vi "Init Command Data.vi"() -> (1 "LBCB 2 Command Data":T1, 2 "LBCB 1 Command Data":T1)   [LabVIEW 2013]
uses:
  MixedMode/Target Data.ctl
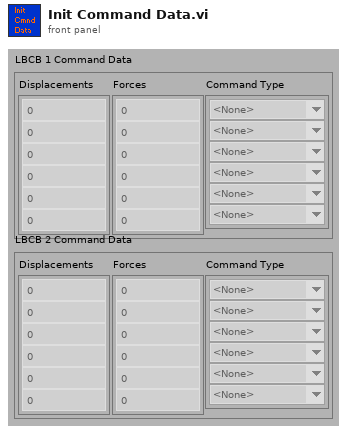
[diagram p1: front panel]
types:
  T1 = typedef "Target Data.ctl" = cluster{"Displacements":dbl[], "Command Type":enum16{"<None>", "Displacement", "Force"}[], "Forces":dbl[]}
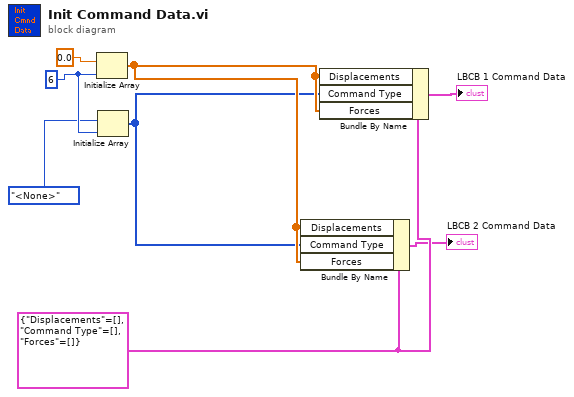
[diagram p0: block diagram]
diagram:
  w7 = 6 ("dimension size")
  w6 = T1 {"Displacements"=[], "Command Type"=[], "Forces"=[]} ("LBCB 1 Command Data")
  n1 = Initialize Array(0.0, w7) -> (w3:dbl[])
  n2 = Initialize Array(enum16{"<None>", "Displacement", "Force"}."<None>" ("Enum"), w7) -> (w2:enum16{"<None>", "Displacement", "Force"}[])
  n3 = Bundle By Name(cluster=w6, "Displacements"=w3, "Command Type"=w2, "Forces"=w3) -> (→"LBCB 2 Command Data":T1)
  n4 = Bundle By Name(cluster=w6, "Displacements"=w3, "Command Type"=w2, "Forces"=w3) -> (→"LBCB 1 Command Data":T1)
